vi "Close.vi"(8 "error in (no error)":errorcluster, 11 "hDevice":i32) -> (0 "error out":errorcluster)   [LabVIEW 2011, in "Thorlabs_MDT69xB.lvlib"]
doc: "Performs an instrument error query before terminating the software connection to the instrument."
uses:
  <instrlib>/Thorlabs_MDT69xB/Thorlabs_MDT69xB.lvlib
  <instrlib>/Thorlabs_MDT69xB/Data/MDT_COMMAND_LIB_win32.dll
  <instrlib>/Thorlabs_MDT69xB/Data/MDT_COMMAND_LIB_x64.dll
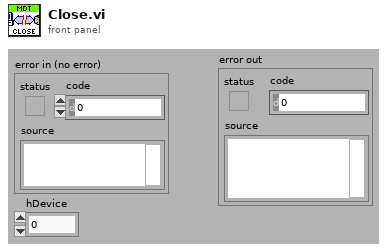
[diagram p1: front panel]
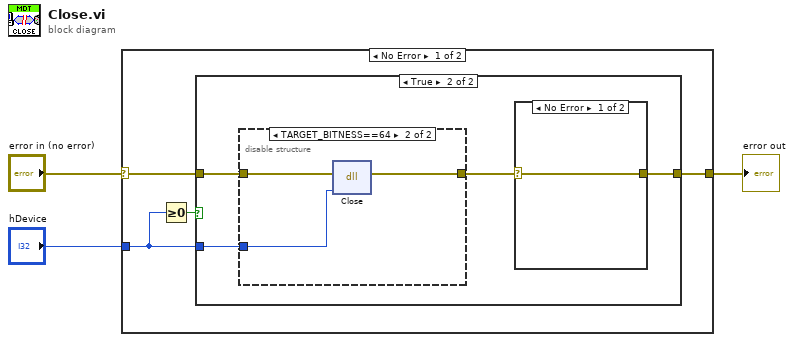
[diagram p0: block diagram]
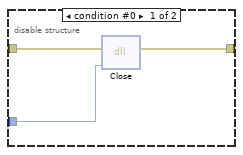
[diagram p3: hidden frame]
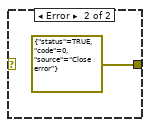
[diagram p4: hidden frame]
diagram:
  n1 = case shown="No Error" "error in (no error)" {
    selector: "error in (no error)" -> [w7 w21]
    tunnel: "hDevice" -> [w4 _]
    tunnel: [w6 w21] -> w1
    frame No Error {
      n2 = Greater Or Equal To 0?(x=w4) -> (x >= 0?=w5:bool)
      n3 = case shown="True" w5 {
        tunnel: w7 -> [w8 w11]
        tunnel: w4 -> [_ w9]
        tunnel: [w8 w12] -> w6
        frame False {
        }
        frame True {
          n4 = disable-structure shown="TARGET_BITNESS==64" {
            disable-tunnel: w11 -> [w15 w18]
            disable-tunnel: [w14 w17] -> w10
            disable-tunnel: w9 -> [w13 w16]
            frame condition #0 {
              n5 = dll-call lib="E:/Program Files (x86)/National Instruments/LabVIEW 2011/instr.lib/Thorlabs_MDT69xB/Data/MDT_COMMAND_LIB_win32.dll" fn="Close"(error in=w15, "hdl"=w13) -> (error out=w14:errorcluster)  [unwired: 4 in, 1 out]
            }
            frame condition #1 (active) {
              n6 = dll-call lib="D:/Program Files/National Instruments/LabVIEW 2011/instr.lib/Thorlabs_MDT69xB/Data/MDT_COMMAND_LIB_x64.dll" fn="Close"(error in=w18, "hdl"=w16) -> (error out=w17:errorcluster)  [unwired: 4 in, 1 out]
            }
          }
          n7 = case shown="No Error" w10 {
            selector: w10 -> [w19 _]
            tunnel: [w19 errorcluster {"status"=TRUE, "code"=0, "source"="Close error"} ("error out")] -> w12
            frame No Error {
            }
            frame Error {
            }
          }
        }
      }
    }
    frame Error {
    }
  }
  "error out" <- w1
